vi "Convert Ticks to msecs.vi"(9 "Division":u16, 10 "ms/b":u32, 11 "Delta Time":u32) -> (3 "Delta Time msec":u32)   [LabVIEW 2016]
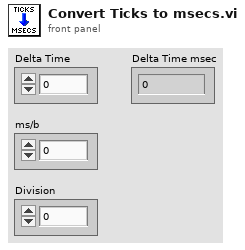
[diagram p1: front panel]
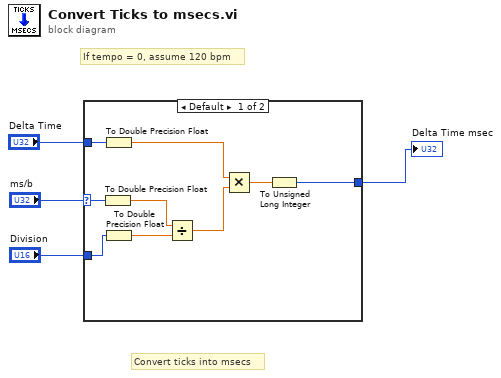
[diagram p0: block diagram]
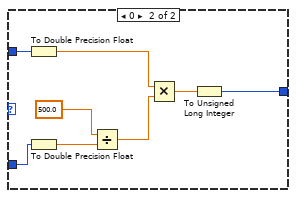
[diagram p2: hidden frame]
diagram:
  # "Convert ticks into msecs"
  # "If tempo = 0, assume 120 bpm"
  n1 = case shown="Default" "ms/b" {
    selector: "ms/b" -> [w13 _]
    tunnel: "Division" -> [w12 w21]
    tunnel: "Delta Time" -> [w11 w20]
    tunnel: [w5 w15] -> w1
    frame Default {
      n2 = To Double Precision Float(number=w13) -> (double precision float=w7:dbl)
      n3 = To Double Precision Float(number=w11) -> (double precision float=w8:dbl)
      n4 = To Double Precision Float(number=w12) -> (double precision float=w6:dbl)
      n5 = Divide(x=w7, y=w6) -> (x/y=w10:dbl)
      n6 = Multiply(x=w8, y=w10) -> (x*y=w9:dbl)
      n7 = To Unsigned Long Integer(number=w9) -> (unsigned 32bit integer=w5:u32)
    }
    frame 0 {
      n8 = To Double Precision Float(number=w20) -> (double precision float=w17:dbl)
      n9 = To Double Precision Float(number=w21) -> (double precision float=w16:dbl)
      n10 = Divide(x=500.0, y=w16) -> (x/y=w19:dbl)
      n11 = Multiply(x=w17, y=w19) -> (x*y=w18:dbl)
      n12 = To Unsigned Long Integer(number=w18) -> (unsigned 32bit integer=w15:u32)
    }
  }
  "Delta Time msec" <- w1
